vi "Setup Enable Data.vi"(8 "Error":errorcluster, 11 "FP":refnum<class "DecFrame_FP.lvclass">) -> (0 "Error Out":errorcluster, 3 "FP Out":refnum<class "DecFrame_FP.lvclass">)   [LabVIEW 2024, in "DecFrame_FP.lvclass"]
uses:
  DecFrame_FP.lvclass
  DecFrame_FP.lvclass/DecFrame_FP.ctl
  TypeDefs_Utility/Cluster_FP_Scroll Bars Hide Show.ctl
  TypeDefs_Utility/ENUM_FP_Show-Hide Select.ctl
  TypeDefs_Utility/Cluster_FP_Show Hide Items.ctl
  FPEN/FPEN.lvclass
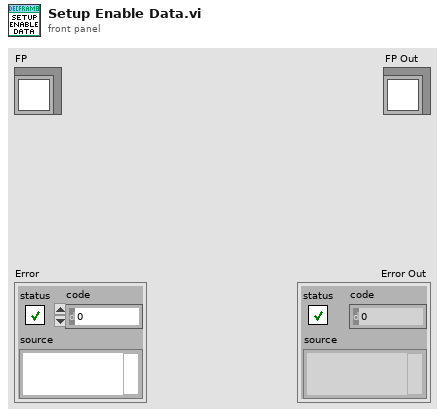
[diagram p1: front panel]
types:
  T1 = typedef "Cluster_FP_Show Hide Items.ctl" = cluster{"MenuBar":T2, "FreeRunButton":T2, "RunButton":T2, "AbortButton":T2, "ToolBar":T2, "Resize":T2, "Closeable":T2, "Minimizable":T2}
  T2 = typedef "ENUM_FP_Show-Hide Select.ctl" = enum16{"No Change", "Hide", "Show"}
  T3 = typedef "Cluster_FP_Scroll Bars Hide Show.ctl" = cluster{"Horiz SBar":T2, "Vert SBar":T2}
  T4 = enum32{"invalid app kind", "Development System", "Run Time System", "Student Edition", "Embedded LabVIEW", "Evaluation", "Custom"}
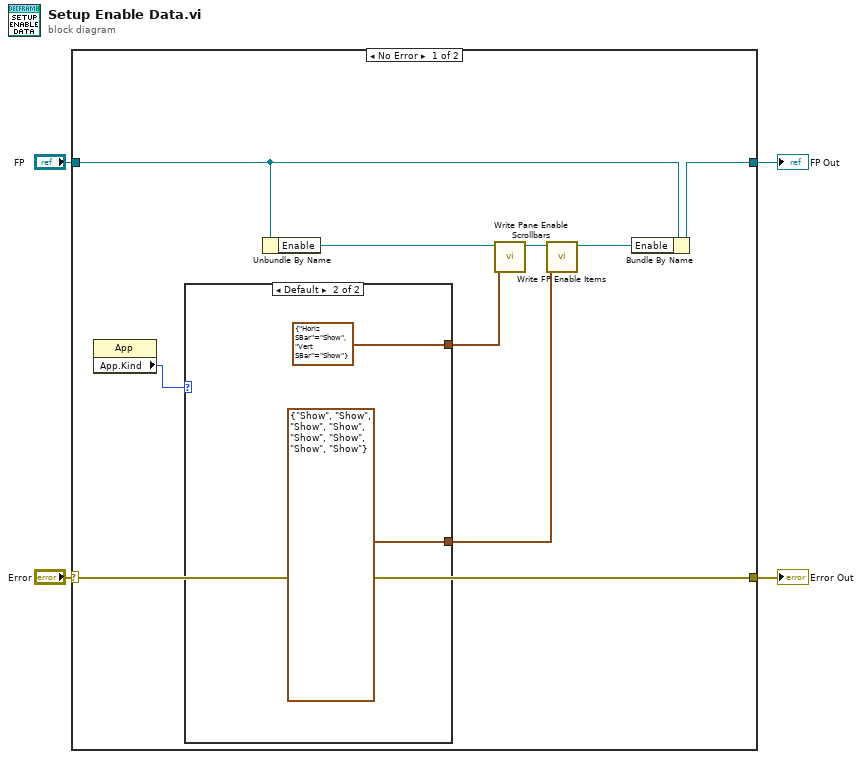
[diagram p0: block diagram]
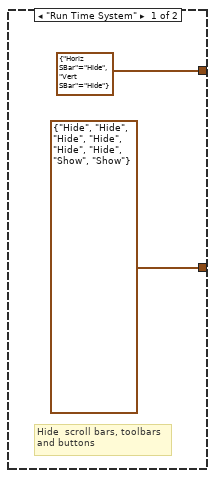
[diagram p2: hidden frame]
diagram:
  n1 = case shown="No Error" "Error" {
    selector: "Error" -> [w6 w19]
    tunnel: [w6 w19] -> w3
    tunnel: [w12 w18] -> w1
    tunnel: "FP" -> [w13 w18]
    frame No Error {
      n2 = property class="App"() -> ("App.Kind"=w5:T4)  [unwired: 2 in, 2 out]
      n3 = case shown="Default" w5 {
        tunnel: [T3 {"Horiz SBar"=enum."Hide", "Vert SBar"=enum."Hide"} ("Scrollbar Settings") T3 {"Horiz SBar"=enum."Show", "Vert SBar"=enum."Show"} ("Scrollbar Settings")] -> w11
        tunnel: [T1 {"MenuBar"=enum."Hide", "FreeRunButton"=enum."Hide", "RunButton"=enum."Hide", "AbortButton"=enum."Hide", "ToolBar"=enum."Hide", "Resize"=enum."Hide", "Closeable"=enum."Show", "Minimizable"=enum."Show"} ("FP Show Hide") T1 {"MenuBar"=enum."Show", "FreeRunButton"=enum."Show", "RunButton"=enum."Show", "AbortButton"=enum."Show", "ToolBar"=enum."Show", "Resize"=enum."Show", "Closeable"=enum."Show", "Minimizable"=enum."Show"} ("FP Show Hide")] -> w10
        frame "Run Time System" {
          # "Hide  scroll bars, toolbars\nand buttons"
        }
        frame Default {
        }
      }
      n4 = Unbundle By Name(w13) -> ("Enable"=w8:refnum<class "FPEN.lvclass">)
      n5 = call "Write Pane Enable Scrollbars.vi"("Pane"=w11, "FPEN"=w8) -> ("FPEN Out"=w9:refnum<class "FPEN.lvclass">)  [unwired: 9 in]
      n6 = call "Write FP Enable Items.vi"("FP Enable Items"=w10, "FPEN"=w9) -> ("FPEN Out"=w7:refnum<class "FPEN.lvclass">)  [unwired: 9 in]
      n7 = Bundle By Name(cluster=w13, "Enable"=w7) -> (w12:refnum<class "DecFrame_FP.lvclass">)
    }
    frame Error {
    }
  }
  "Error Out" <- w3
  "FP Out" <- w1
